vi "InitMagnetInterface.vi"(8 "error in (no error)":errorcluster) -> (0 "error out":errorcluster, 3 "output cluster 2":T1={"Main interlock"=TRUE, "Flow Switch 1"=TRUE, "Flow Switch 2"=TRUE, "Power Supply ok"=FALSE, "on"=TRUE, "staging"=TRUE, "undulator"=FALSE, "VOLTAGE"=0.0, "CURRENT"=0.0, "curent set"=0})   [LabVIEW 2013]
uses:
  MagnetCluster.ctl
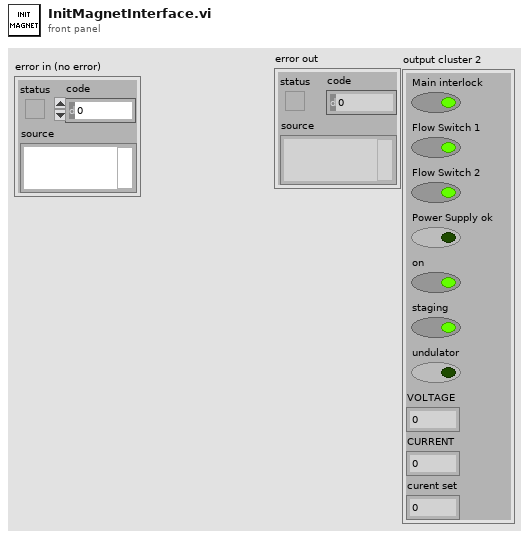
[diagram p1: front panel]
types:
  T1 = typedef "MagnetCluster.ctl" = cluster{"Main interlock":bool, "Flow Switch 1":bool, "Flow Switch 2":bool, "Power Supply ok":bool, "on":bool, "staging":bool, "undulator":bool, "VOLTAGE":dbl, "CURRENT":dbl, "curent set":u16}
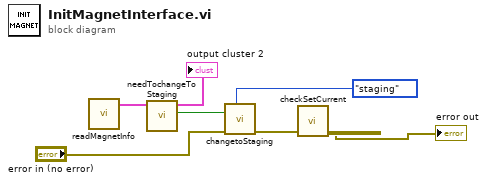
[diagram p0: block diagram]
diagram:
  n1 = call "readMagnetInfo.vi"() -> ("output cluster"=w7:T1)  [unwired: 10 in, 1 out]
  n2 = call "needTochangeToStaging.vi"("output cluster"=w7) -> ("change to staging"=w6:bool, "output cluster 2"=→"output cluster 2":T1)  [unwired: 9 in]
  n3 = call "changetoStaging.vi"("cmd"=enum16{"off", "on", "undulator", "staging"}."staging", "error in (no error)"="error in (no error)", "send (true)"=w6) -> ("error out"=w2:errorcluster)  [unwired: 8 in]
  n4 = call "checkSetCurrent.vi"("error in (no error)"=w2) -> ("DS read error"=→"error out":errorcluster)  [unwired: 10 in]
